vi "Initial.vi"(7 "Serial Configuration":T1={"Baud Rate"=9600, "Parity"=0, "Stop Bits"=10, "Flow Control"=2} {"Flow Control" items=["None", "XON/XOFF", "RTS/CTS", "XON/XOFF & RTS/CTS", "DTR/DSR", "XON/XOFF & DTR/DSR"]; "Stop Bits" items=["1.0"=10, "1.5"=15, "2.0"=20]; "Parity" items=["None", "Odd", "Even", "Mark", "Space"]; "Baud Rate" items=["300"=300, "600"=600, "1200"=1200, "2400"=2400, "4800"=4800, "9600"=9600, "19200"=19200]}, 8 "error in (no error)":errorcluster, 9 "ID Query? (T: Yes)":bool=TRUE, 10 "Reset? (T: Yes)":bool=TRUE, 11 "Tektonix 2000 in":refnum<class "Tektonix 2000.lvclass">) -> (0 "error out":errorcluster, 3 "reference out":refnum<class "Tektonix 2000.lvclass">)   [LabVIEW 2020, in "Osciloscope Tektronix.lvlib" / "Tektonix 2000.lvclass"]
uses:
  Tektonix 2000.lvclass
  C:/Users/Pablo/Osciloscope-Tek/TDS2000/Libraries/Osciloscope Tektronix/Clases/Osciloscope/Osciloscope.lvclass
  Osciloscope/Osciloscope.lvclass/Osciloscope.ctl
  Osciloscope/Read COM.vi
  <instrlib>/Tektronix TDS 200 1000 2000 Series/Tektronix TDS 200 1000 2000 Series.lvlib
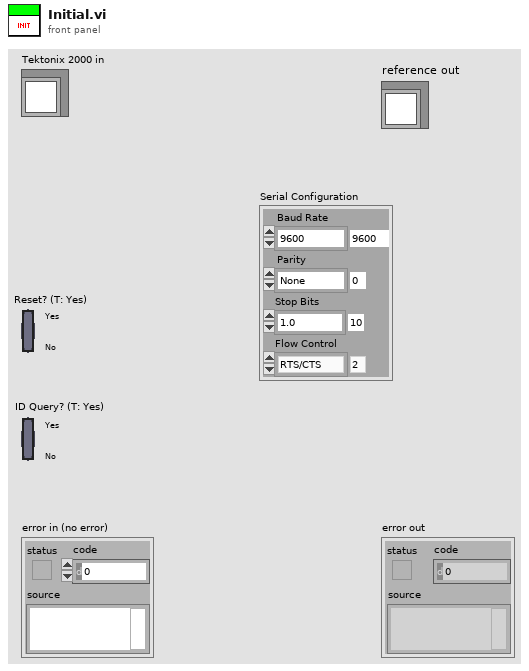
[diagram p1: front panel]
types:
  T1 = cluster{"Baud Rate":u32, "Parity":u16, "Stop Bits":u16, "Flow Control":u16}
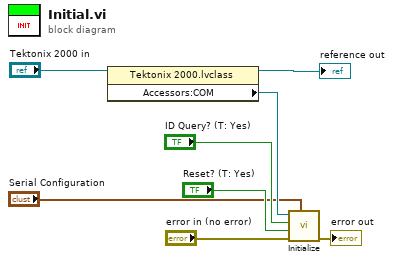
[diagram p0: block diagram]
diagram:
  n1 = property class="Tektonix 2000.lvclass"(reference="Tektonix 2000 in") -> (reference out=→"reference out":refnum<class "Tektonix 2000.lvclass">, "Accessors:COM"=w7:refnum<visa-resource-name>)  [unwired: 1 in, 1 out]
  n2 = call <instrlib>:"Initialize.vi"("Serial Configuration"="Serial Configuration", "error in (no error)"="error in (no error)", "Reset? (T: Yes)"="Reset? (T: Yes)", "ID Query? (T: Yes)"="ID Query? (T: Yes)", "VISA resource name"=w7) -> ("error out"=→"error out":errorcluster)  [unwired: 5 in, 1 out]
